vi "Extraction - Send to JMP.vi"(7 "Send to JMP":bool, 8 "Error In":errorcluster, 11 "filename":string="C:\\Users\\niko.kuusniemi\\Documents\\Python Scripts\\new\\_Extraction.csv") -> (0 "Error Out":errorcluster)   [LabVIEW 2020]
uses:
  <vilib>/Utility/file.llb/Read Delimited Spreadsheet (string).vi
panel:
  out "FullName":string
  out "Path":string
  out "size(s)":i32
  in  "JMP.IJMPAutoApp":refnum<k7>
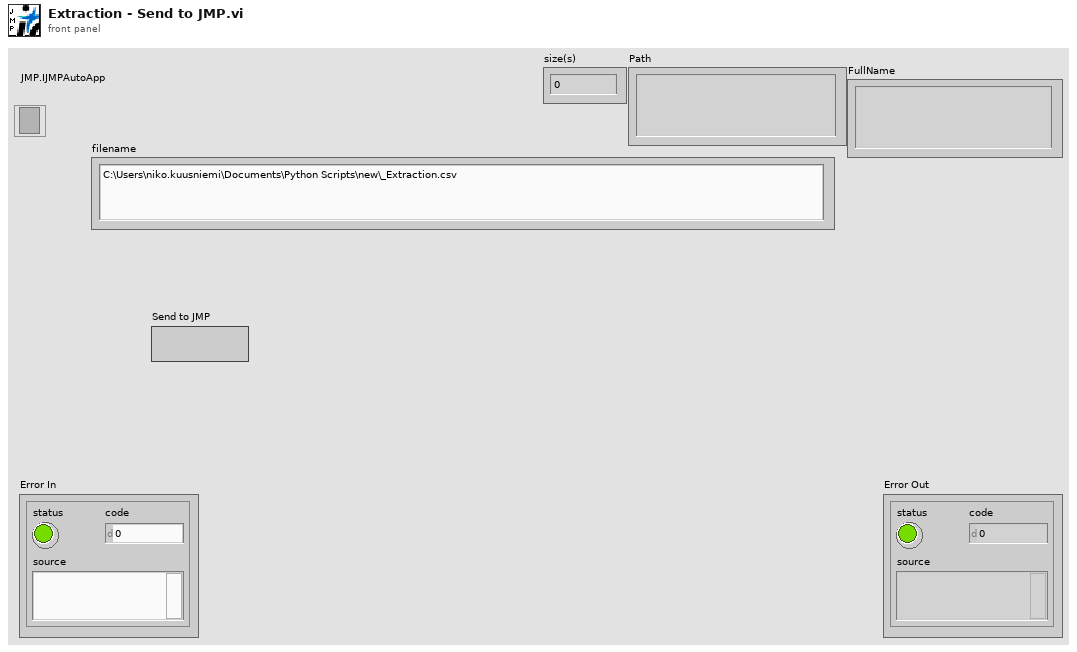
[diagram p1: front panel]
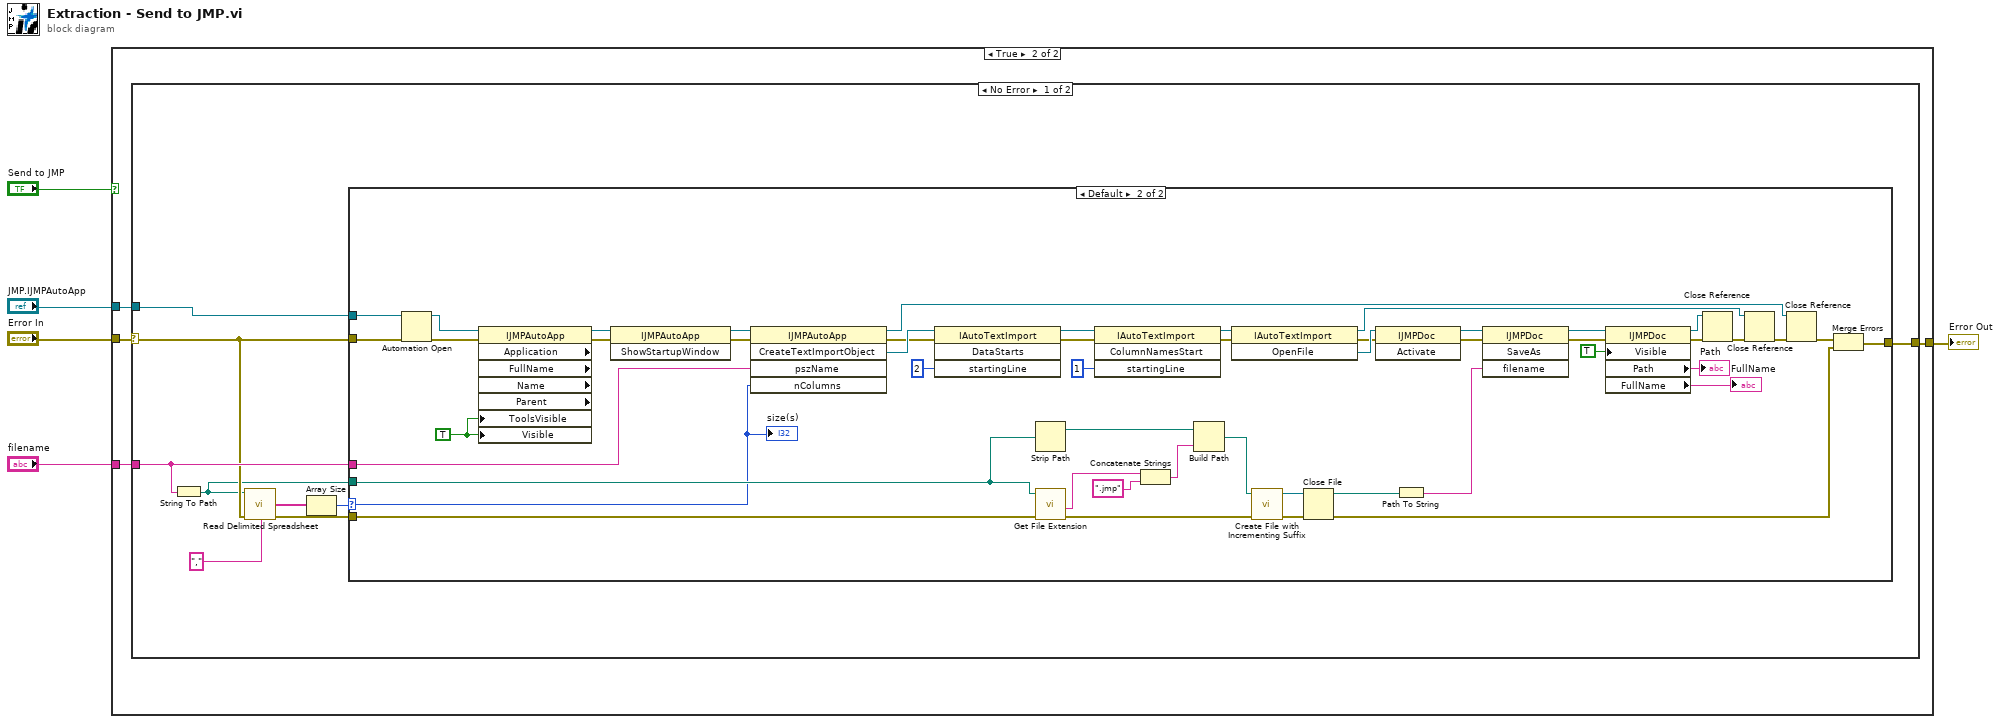
[diagram p0: block diagram]
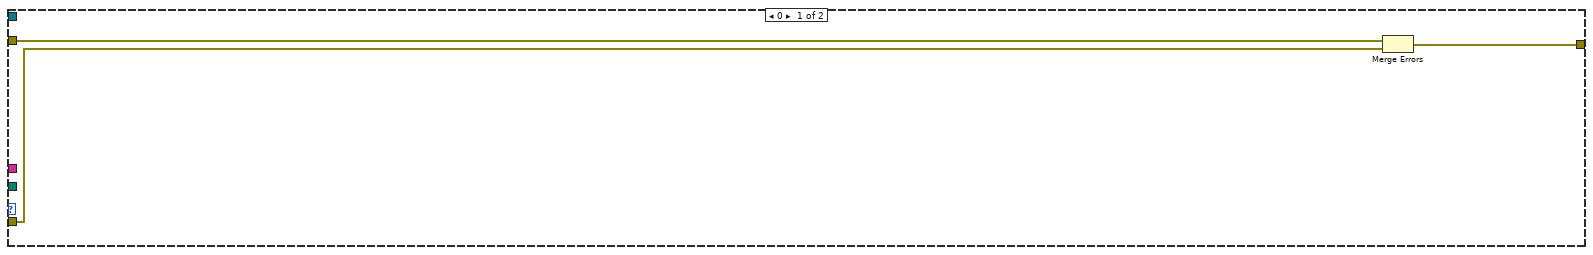
[diagram p3: hidden frame]
diagram:
  n1 = case shown="True" "Send to JMP" {
    tunnel: "JMP.IJMPAutoApp" -> [_ w10]
    tunnel: "filename" -> [_ w9]
    tunnel: "Error In" -> [w6 w8]
    tunnel: [w6 w7] -> w2
    frame False {
    }
    frame True {
      n2 = case shown="No Error" w8 {
        selector: w8 -> [w15 w72]
        tunnel: w10 -> [w19 _]
        tunnel: w9 -> [w18 _]
        tunnel: [w14 w72] -> w7
        frame No Error {
          n3 = String To Path(string=w18) -> (path=w13:path)
          n4 = call-poly <vilib>:"Read Delimited Spreadsheet.vi"("file path (dialog if empty)"=w13, "error in (no error)"=w15, "delimiter (\\t)"="," ("delimiter (\\t)")) -> ("first row"=w16:string[], "error out"=w12:errorcluster)  [unwired: 7 in, 4 out]
          n5 = Array Size(array=w16) -> (size(s)=w11:i32)
          n6 = case shown="Default" w11 {
            selector: w11 -> [_ w29]
            tunnel: w19 -> [_ w70]
            tunnel: w18 -> [_ w50]
            tunnel: w15 -> [w22 w49]
            tunnel: [w20 w47] -> w14
            tunnel: w13 -> [_ w41]
            tunnel: w12 -> [w21 w31]
            frame 0 {
              n7 = Merge Errors(w22, w21) -> (w20:errorcluster)
            }
            frame Default {
              w51 = TRUE ("Visible")
              n8 = Automation Open(error in (no error)=w49, Automation Refnum=w70) -> (Automation Refnum=w71:refnum<k7>, error out=w56:errorcluster)  [unwired: 2 in]
              n9 = property class="IJMPAutoApp" props=["Application", "FullName", "Name", "Parent", "ToolsVisible", "Visible"](reference=w71, error in=w56, "ToolsVisible"=w51, "Visible"=w51) -> (reference out=w46:refnum<k7>, error out=w44:errorcluster)  [unwired: 4 out]
              n10 = invoke class="IJMPAutoApp" method="ShowStartupWindow"(reference=w46, error in=w44) -> (reference out=w45:refnum<k7>, error out=w43:errorcluster)  [unwired: 1 in, 1 out]
              n11 = invoke class="IJMPAutoApp" method="CreateTextImportObject"(reference=w45, error in=w43, "pszName"=w50, "nColumns"=w29) -> (reference out=w66:refnum<k7>, error out=w59:errorcluster, "CreateTextImportObject"=w60:refnum<k7>)  [unwired: 1 in, 2 out]
              n12 = invoke class="IAutoTextImport" method="DataStarts"(reference=w60, error in=w59, "startingLine"=2) -> (reference out=w64:refnum<k7>, error out=w63:errorcluster)  [unwired: 1 in, 2 out]
              n13 = Strip Path(path=w41) -> (stripped path=w40:path)  [unwired: 1 out]
              n14 = call <vilib>:"Get File Extension.vi"("error in (no error)"=w31, "file"=w41) -> ("error out"=w23:errorcluster, "filename without extension"=w39:string)  [unwired: 5 in, 3 out]
              n15 = invoke class="IAutoTextImport" method="ColumnNamesStart"(reference=w64, error in=w63, "startingLine"=1) -> (reference out=w62:refnum<k7>, error out=w61:errorcluster)  [unwired: 1 in, 2 out]
              n16 = Concatenate Strings(w39, ".jmp" ("string")) -> (w38:string)
              n17 = Build Path(base path=w40, name or relative path=w38) -> (appended path=w28:path)
              n18 = invoke class="IAutoTextImport" method="OpenFile"(reference=w62, error in=w61) -> (reference out=w68:refnum<k7>, error out=w55:errorcluster, "OpenFile"=w65:refnum<k7>)  [unwired: 1 in]
              n19 = call <vilib>:"Create File with Incrementing Suffix.vi"("error in (no error)"=w23, "file path"=w28) -> ("error out"=w24:errorcluster, "refnum out"=w27:refnum<file>)  [unwired: 7 in, 1 out]
              n20 = Close File(refnum=w27, error in=w24) -> (path=w26:path, error out=w25:errorcluster)
              n21 = invoke class="IJMPDoc" method="Activate"(reference=w65, error in=w55) -> (reference out=w35:refnum<k7>, error out=w33:errorcluster)  [unwired: 1 in, 1 out]
              n22 = Path To String(path=w26) -> (string=w36:string)
              n23 = invoke class="IJMPDoc" method="SaveAs"(reference=w35, error in=w33, "filename"=w36) -> (reference out=w34:refnum<k7>, error out=w32:errorcluster)  [unwired: 1 in, 2 out]
              n24 = property class="IJMPDoc"(reference=w34, error in=w32, "Visible"=TRUE) -> (reference out=w52:refnum<k7>, error out=w53:errorcluster, "Path"=→"Path":string, "FullName"=→"FullName":string)
              n25 = Close Reference(reference=w52, error in (no error)=w53) -> (error out=w69:errorcluster)
              n26 = Close Reference(reference=w68, error in (no error)=w69) -> (error out=w67:errorcluster)
              n27 = Close Reference(reference=w66, error in (no error)=w67) -> (error out=w48:errorcluster)
              n28 = Merge Errors(w48, w25) -> (w47:errorcluster)
              "size(s)" <- w29
            }
          }
        }
        frame Error {
        }
      }
    }
  }
  "Error Out" <- w2
